vi "Light fade.vi"(10 "rate pf change":dbl=1.0 format="%#_13g", 11 "value":dbl) -> (3 "Output":dbl)   [LabVIEW 2014]
uses:
  <vilib>/ptbypt/NI_PtbyPt.lvlib
panel:
  out "Old value":dbl
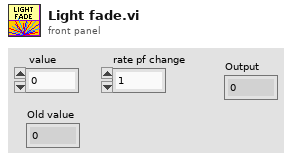
[diagram p1: front panel]
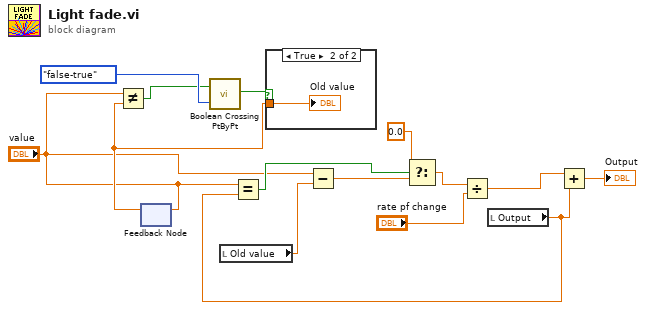
[diagram p0: block diagram]
diagram:
  n1 = feedback #1() -> (w13:dbl)  [unwired: 1 in]
  n2 = Not Equal?(x="value", y=w13) -> (x != y?=w7:bool)
  n3 = feedback-in #1("value") -> ()
  n4 = call <vilib>:"Boolean Crossing PtByPt.vi"("direction"=enum16{"either", "false-true", "true-false"}."false-true", "input"=w7) -> ("crossing"=w11:bool)  [unwired: 1 in]
  n5 = local read "Old value"() -> (w8:dbl)
  n6 = case shown="True" w11 {
    tunnel: w13 -> [_ w15]
    frame False {
    }
    frame True {
      "Old value" <- w15
    }
  }
  n7 = Subtract(x="value", y=w8) -> (x-y=w2:dbl)
  n8 = local read "Output"() -> (w5:dbl)
  n9 = Equal?(x="value", y=w5) -> (x = y?=w6:bool)
  n10 = Select(t=0.0, s=w6, f=w2) -> (s? t:f=w1:dbl)
  n11 = Divide(x=w1, y="rate pf change") -> (x/y=w10:dbl)
  n12 = Add(x=w10, y=w5) -> (x+y=→"Output":dbl)
